vi "Control Panel No Objects.vi"(8 "error in (no error)":errorcluster) -> (0 "error out":errorcluster)   [LabVIEW 2009]
doc: "(Dynamic) A user-level application that simulates the physical front panel of the Instrument. Provide the user with buttons to manually control features of the instrument, and provide indicators of its current state."
uses:
  Global/GPIB Numbers.vi
  Microwave Amp/MicrowaveAmplifier.lvlib
panel:
  in  "Copy actual to set":bool
  in  "Populate fields with member data":bool
  in  "Read Remaining Time Delay":bool
  in  "Read Amplifier Status/Mode":bool
  in  "Standby":bool
  in  "stop":bool
  out "Mode":u16(ring) items=["SLEEP", "WARM-UP", "STANDBY", "OPERATE", "FAULT"]
  in  "Operate":bool
  in  "Read Reverse Power Out (W)":bool
  in  "Read Reverse Power Out (dBm)":bool
  in  "Read Forward Power Out (W)":bool
  in  "Read Forward Power out (dBm)":bool
  in  "Read Gain":bool
  in  "Set Gain":bool
  out "Remaining Heater Delay Time":dbl[unit]
  out "Reverse Power Out (dBm)":dbl
  out "Reverse Power Out (W)":dbl[unit]
  out "Forward Power Out (dBm)":dbl
  out "Forward Power Out (W)":dbl[unit]
  out "Gain (%)":dbl
  in  "GainSet":dbl
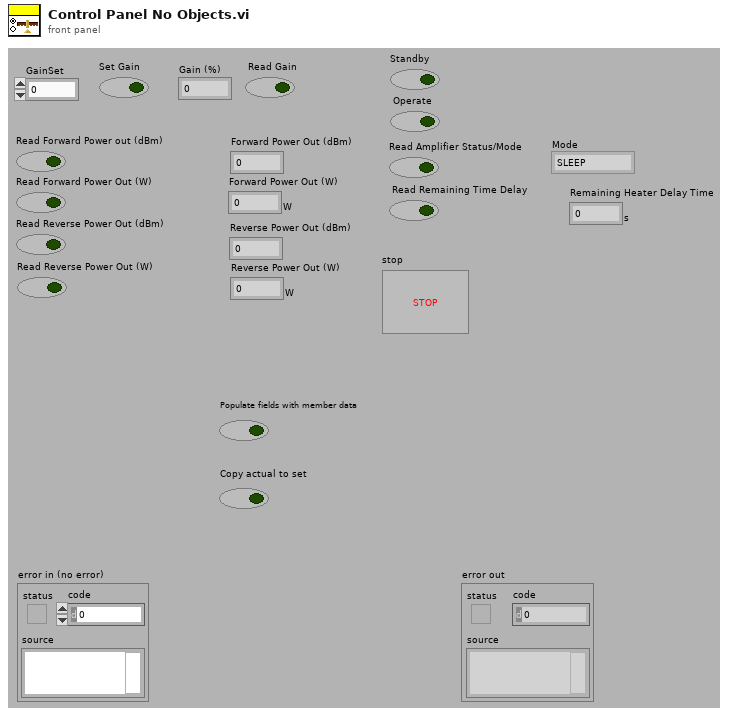
[diagram p1: front panel]
types:
  T1 = cluster{"Gain (%)":dbl, "Forward Power Out (dBm)":dbl, "Forward Power Out (W)":dbl[unit], "Reverse Power Out (dBm)":dbl, "Reverse Power Out (W)":dbl[unit], "Mode":u16, "Remaining Heater Delay Time (s)":dbl[unit]}
  T2 = typedef "GPIB Type Def.ctl" = cluster{"Name":string, "bus":dbl, "GPIB":dbl, "GPIB as string":string, "byte":i32, "VISA Resource Name":refnum<visa-resource-name>}
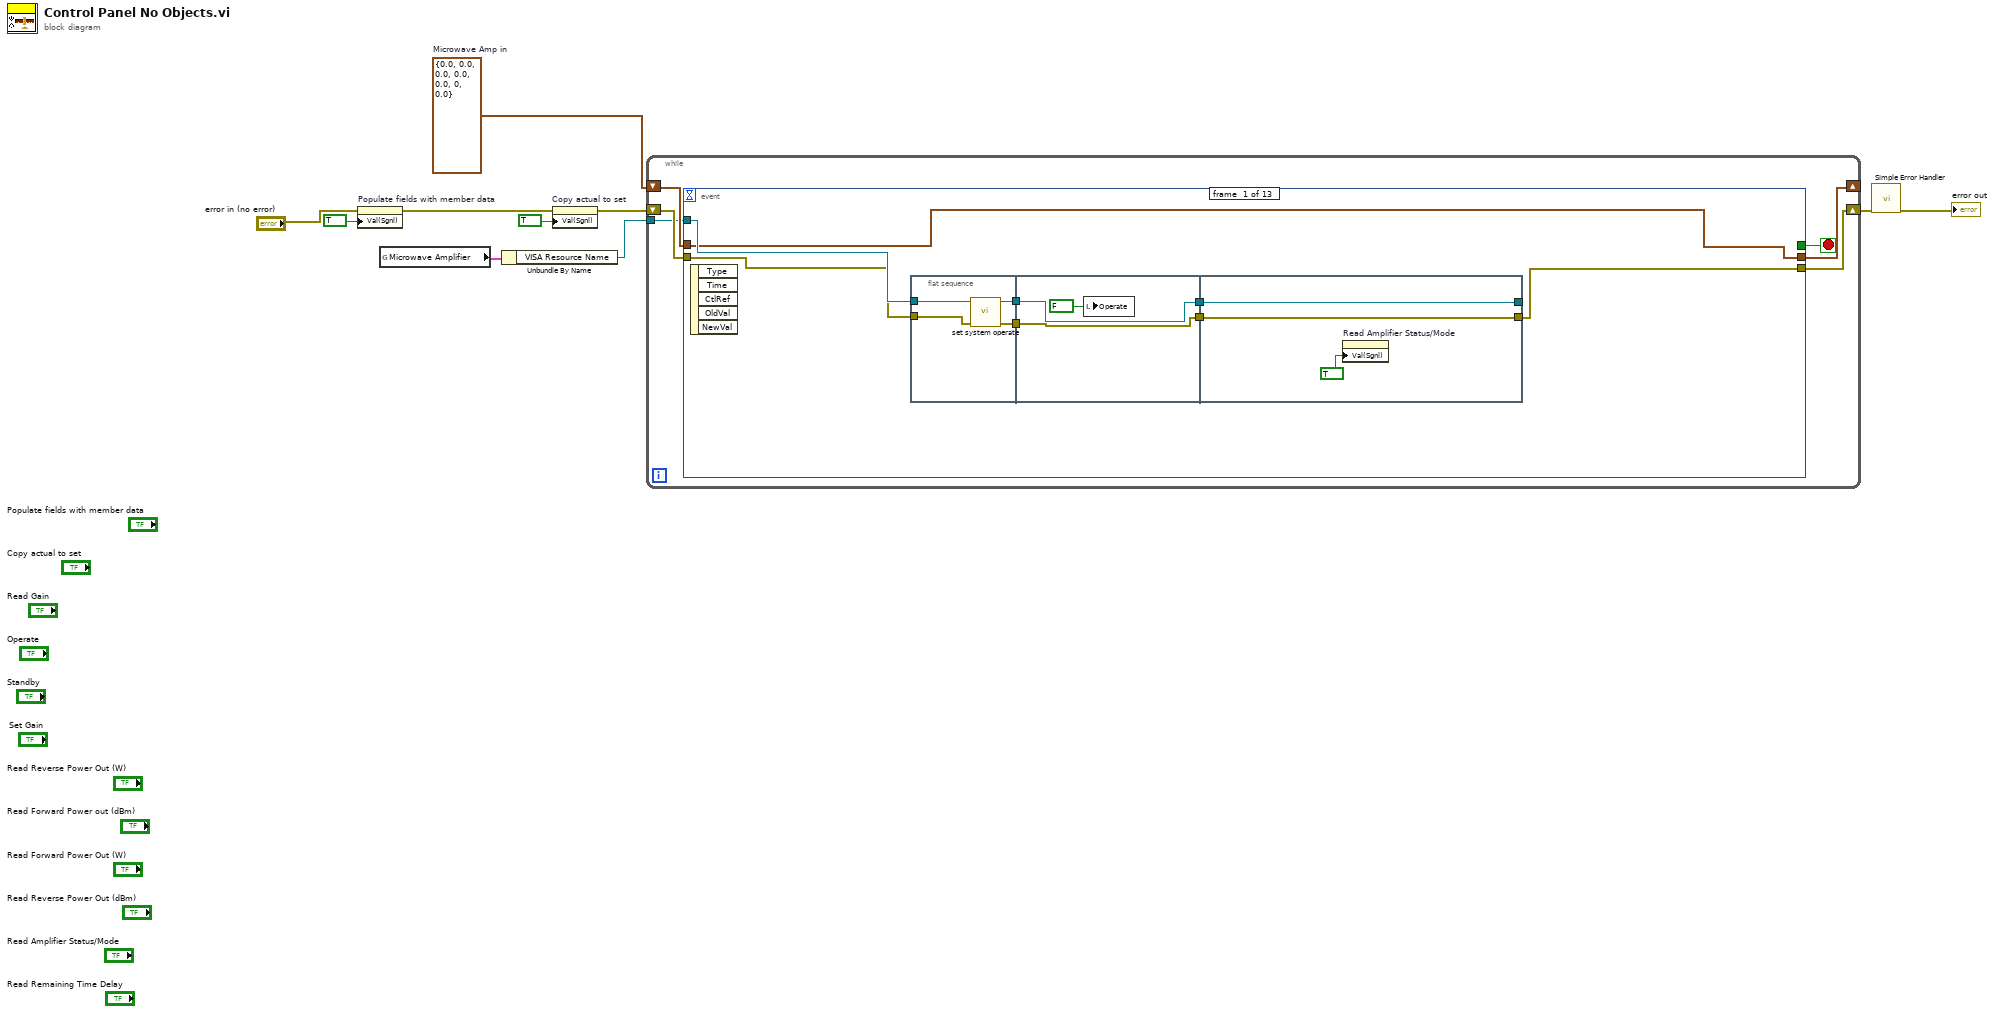
[diagram p0: block diagram]
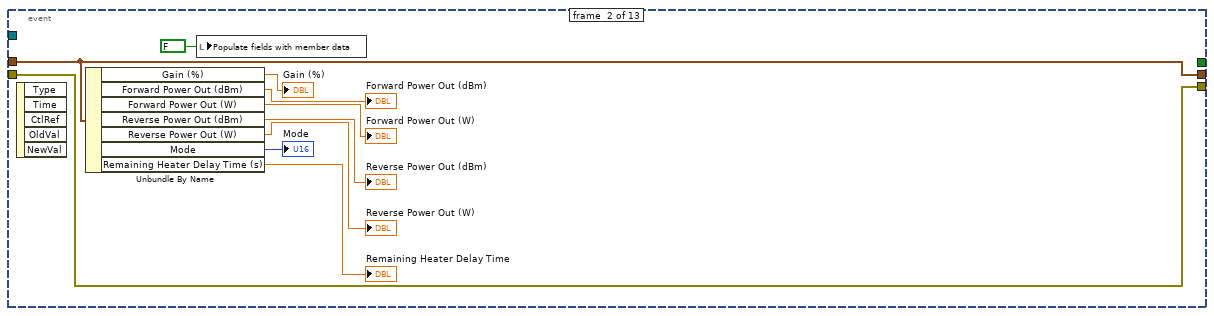
[diagram p2: hidden frame]
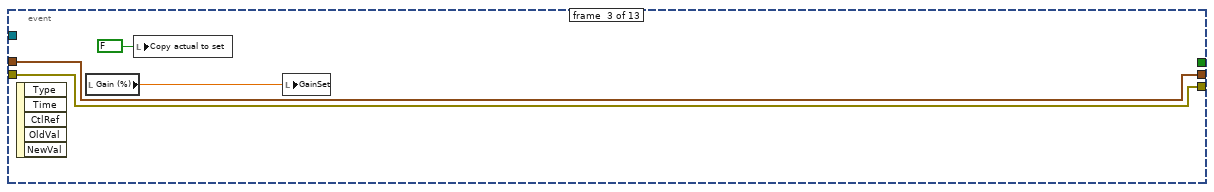
[diagram p3: hidden frame]
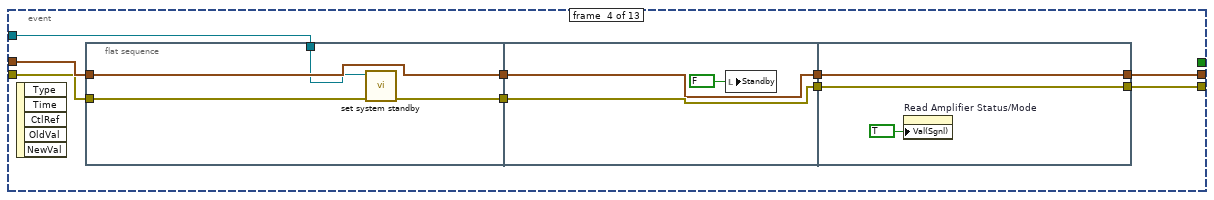
[diagram p4: hidden frame]
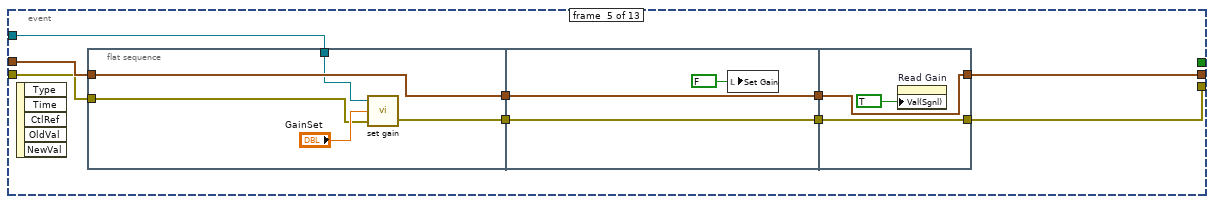
[diagram p5: hidden frame]
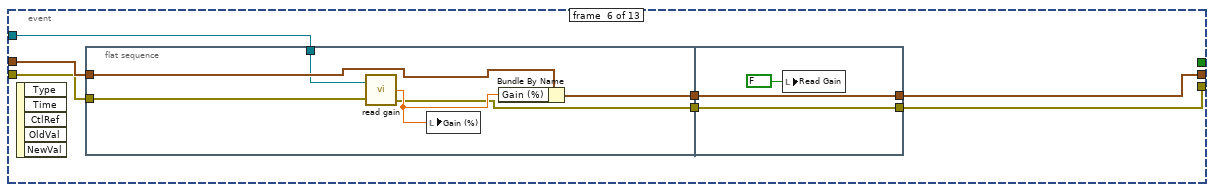
[diagram p6: hidden frame]
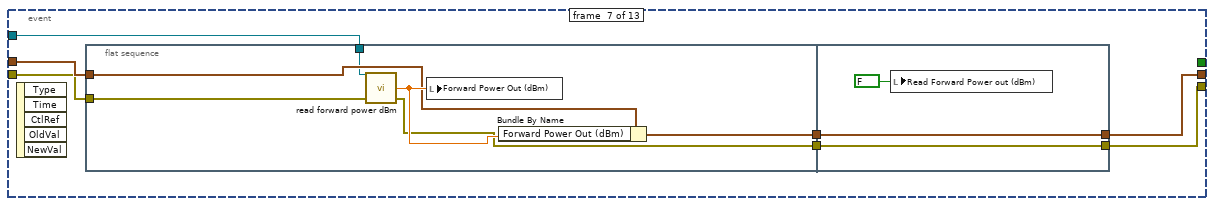
[diagram p7: hidden frame]
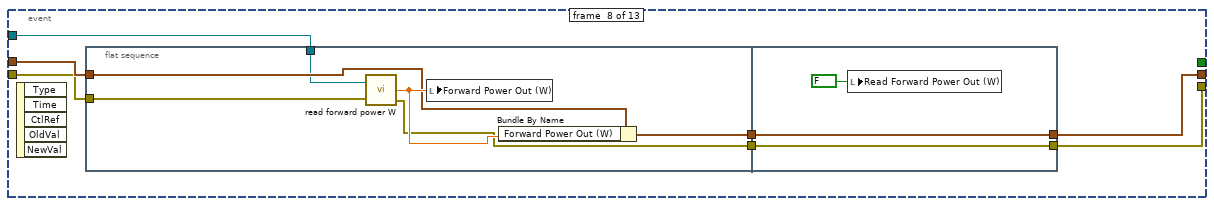
[diagram p8: hidden frame]
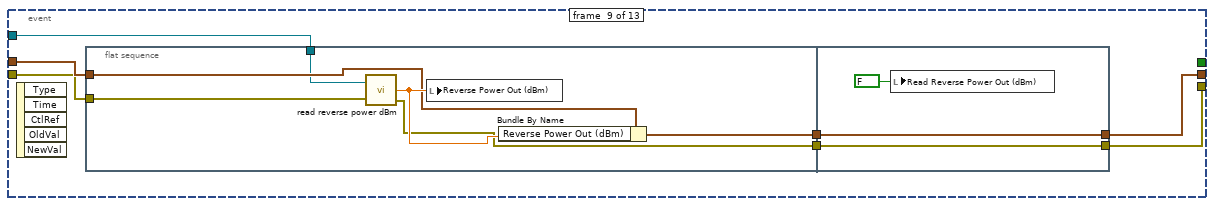
[diagram p9: hidden frame]
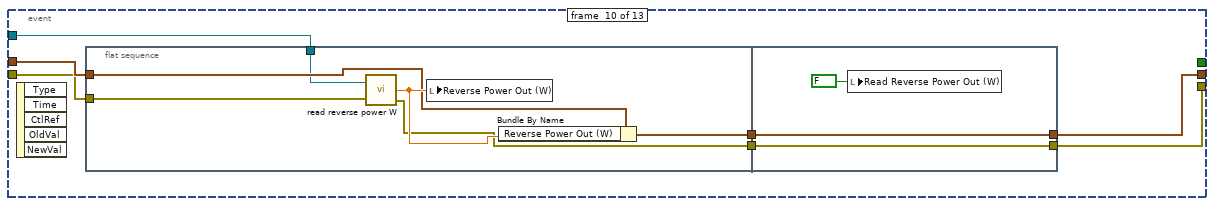
[diagram p10: hidden frame]
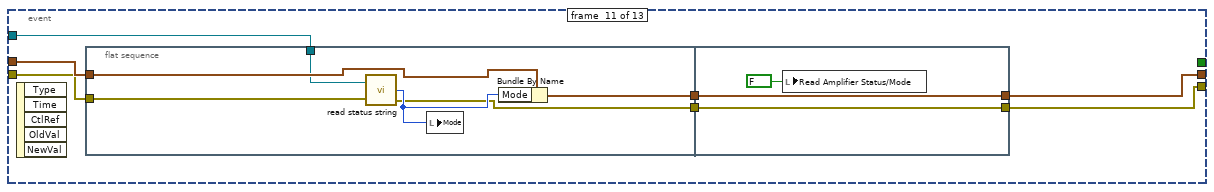
[diagram p11: hidden frame]
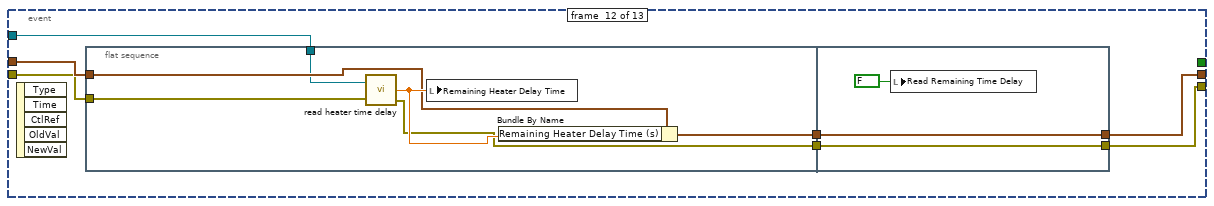
[diagram p12: hidden frame]
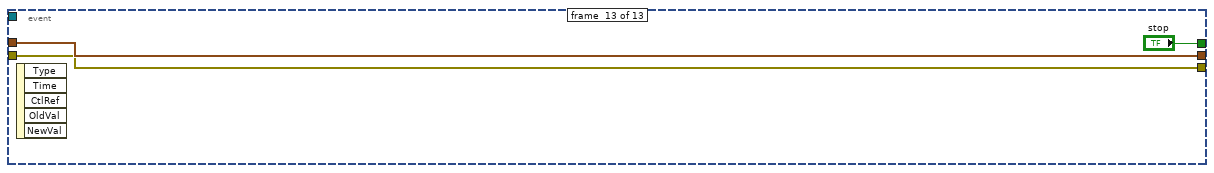
[diagram p13: hidden frame]
diagram:
  w4 = T1 {"Gain (%)"=0.0, "Forward Power Out (dBm)"=0.0, "Forward Power Out (W)"=0.0, "Reverse Power Out (dBm)"=0.0, "Reverse Power Out (W)"=0.0, "Mode"=0, "Remaining Heater Delay Time (s)"=0.0}  # Microwave Amp in
  n1 = property on="Populate fields with member data" class="Bool (strict)"(error in="error in (no error)", "Val(Sgnl)"=TRUE ("Value (Signaling)")) -> (error out=w10:errorcluster)  [unwired: 1 in, 1 out]
  n2 = global read "GPIB Numbers.vi" "Microwave Amplifier"() -> (w2:T2)
  n3 = Unbundle By Name(w2) -> ("VISA Resource Name"=w1:refnum<visa-resource-name>)
  n4 = property on="Copy actual to set" class="Bool (strict)"(error in=w10, "Val(Sgnl)"=TRUE ("Value (Signaling)")) -> (error out=w6:errorcluster)  [unwired: 1 in, 1 out]
  n5 = while {
    shift-right: [w16] -> w9
    shift-left: w6 -> [w13]
    shift-right: [w14] -> _
    shift-left: w4 -> [w12]
    tunnel: w1 -> [w11]
    stop <- w15 stop-if-true
    n6 = event shown="[12] \"stop\": Value Change" {
      selector: _ -> [_ _ _ _ _ _ _ _ _ _ _ _ _]
      dyn-events: _ -> [_ _ _ _ _ _ _ _ _ _ _ _ _]
      timeout: _ -> [_ _ _ _ _ _ _ _ _ _ _ _ _]
      tunnel: w13 -> [w19 w44 w47 w52 w73 w92 w106 w122 w138 w154 w170 w188 w200]
      tunnel: [w17 w44 w47 w56 w69 w89 w105 w121 w137 w153 w169 w185 w200] -> w16
      tunnel: [_ _ _ _ _ _ _ _ _ _ _ _ "stop"] -> w15
      tunnel: w12 -> [w18 w43 w48 w53 w74 w93 w109 w125 w141 w157 w173 w189 w201]
      tunnel: [w18 w43 w48 w54 w72 w91 w108 w124 w140 w156 w172 w187 w201] -> w14
      tunnel: w11 -> [w20 _ _ w49 w68 w88 w104 w120 w136 w152 w168 w184 _]
      event #0 {
        n7 = event-data() -> ()  [unwired: 1 in, 5 out]
        n8 = flat-sequence {
          tunnel: [w28] -> w24
          tunnel: [w27] -> w23
          tunnel: w19 -> [w26]
          tunnel: w20 -> [w25]
          tunnel: w24 -> [w30]
          tunnel: w23 -> [w29]
          tunnel: [w30] -> w22
          tunnel: [w29] -> w21
          tunnel: [w33] -> w17
          tunnel: [w34] -> _
          tunnel: w22 -> [w34]
          tunnel: w21 -> [w33]
          frame #0 {
            n9 = call "set system operate.vi"("error in (no error)"=w26, "VISA resource name"=w25) -> ("error out"=w27:errorcluster, "VISA resource name out"=w28:refnum<visa-resource-name>)  [unwired: 8 in]
          }
          frame #1 {
            n10 = local write "Operate"(FALSE ("Operate")) -> ()
          }
          frame #2 {
            n11 = property on="Read Amplifier Status/Mode" class="Bool (strict)"("Val(Sgnl)"=TRUE ("Value (Signaling)")) -> ()  [unwired: 2 in, 2 out]
          }
        }
      }
      event #1 {
        n12 = event-data() -> ()  [unwired: 1 in, 5 out]
        n13 = Unbundle By Name(w43) -> ("Gain (%)"=→"Gain (%)":dbl, "Forward Power Out (dBm)"=→"Forward Power Out (dBm)":dbl, "Forward Power Out (W)"=→"Forward Power Out (W)":dbl[unit], "Reverse Power Out (dBm)"=→"Reverse Power Out (dBm)":dbl, "Reverse Power Out (W)"=→"Reverse Power Out (W)":dbl[unit], "Mode"=→"Mode":u16, "Remaining Heater Delay Time (s)"=→"Remaining Heater Delay Time":dbl[unit])
        n14 = local write "Populate fields with member data"(FALSE ("Populate fields with member data")) -> ()
      }
      event #2 {
        n15 = event-data() -> ()  [unwired: 1 in, 5 out]
        n16 = local read "Gain (%)"() -> (w45:dbl)
        n17 = local write "Copy actual to set"(FALSE ("Copy actual to set")) -> ()
        n18 = local write "GainSet"(w45) -> ()
      }
      event #3 {
        n19 = event-data() -> ()  [unwired: 1 in, 5 out]
        n20 = flat-sequence {
          tunnel: [w61] -> w57
          tunnel: [w60] -> w55
          tunnel: w53 -> [w60]
          tunnel: w52 -> [w59]
          tunnel: w49 -> [w58]
          tunnel: w57 -> [w63]
          tunnel: w55 -> [w62]
          tunnel: [w63] -> w51
          tunnel: [w62] -> w50
          tunnel: [w66] -> w54
          tunnel: [w67] -> w56
          tunnel: w51 -> [w67]
          tunnel: w50 -> [w66]
          frame #0 {
            n21 = call "set system standby.vi"("error in (no error)"=w59, "VISA resource name"=w58) -> ("error out"=w61:errorcluster)  [unwired: 8 in, 1 out]
          }
          frame #1 {
            n22 = local write "Standby"(FALSE ("Operate")) -> ()
          }
          frame #2 {
            n23 = property on="Read Amplifier Status/Mode" class="Bool (strict)"("Val(Sgnl)"=TRUE ("Value (Signaling)")) -> ()  [unwired: 2 in, 2 out]
          }
        }
      }
      event #4 {
        n24 = event-data() -> ()  [unwired: 1 in, 5 out]
        n25 = flat-sequence {
          tunnel: [w80] -> w76
          tunnel: w74 -> [w79]
          tunnel: w73 -> [w78]
          tunnel: [w79] -> w70
          tunnel: w68 -> [w77]
          tunnel: w76 -> [w83]
          tunnel: [w83] -> w75
          tunnel: [w82] -> w71
          tunnel: w70 -> [w82]
          tunnel: [w87] -> w69
          tunnel: w75 -> [w87]
          tunnel: [w85] -> w72
          tunnel: w71 -> [w85]
          frame #0 {
            n26 = call "set gain.vi"("error in (no error)"=w78, "Gain"="GainSet", "VISA resource name"=w77) -> ("error out"=w80:errorcluster)  [unwired: 1 out]
          }
          frame #1 {
            n27 = local write "Set Gain"(FALSE ("Set Gain")) -> ()
          }
          frame #2 {
            n28 = property on="Read Gain" class="Bool (strict)"("Val(Sgnl)"=TRUE ("Value (Signaling)")) -> ()  [unwired: 2 in, 2 out]
          }
        }
      }
      event #5 {
        n29 = event-data() -> ()  [unwired: 1 in, 5 out]
        n30 = flat-sequence {
          tunnel: [w98] -> w94
          tunnel: w93 -> [w96]
          tunnel: w92 -> [w97]
          tunnel: [w99] -> w90
          tunnel: w88 -> [w95]
          tunnel: [w102] -> w89
          tunnel: w94 -> [w102]
          tunnel: [w101] -> w91
          tunnel: w90 -> [w101]
          frame #0 {
            n31 = call "read gain.vi"("VISA resource name"=w95, "error in (no error)"=w97) -> ("Gain (%)"=w100:dbl, "error out"=w98:errorcluster)  [unwired: 1 out]
            n32 = local write "Gain (%)"(w100) -> ()
            n33 = Bundle By Name(cluster=w96, "Gain (%)"=w100) -> (w99:T1)
          }
          frame #1 {
            n34 = local write "Read Gain"(FALSE ("Read Gain")) -> ()
          }
        }
      }
      event #6 {
        n35 = event-data() -> ()  [unwired: 1 in, 5 out]
        n36 = flat-sequence {
          tunnel: [w112] -> w110
          tunnel: w109 -> [w113]
          tunnel: [w115] -> w107
          tunnel: w106 -> [w114]
          tunnel: w104 -> [w111]
          tunnel: [w119] -> w105
          tunnel: w110 -> [w119]
          tunnel: [w117] -> w108
          tunnel: w107 -> [w117]
          frame #0 {
            n37 = call "read forward power dBm.vi"("error in (no error)"=w114, "VISA resource name"=w111) -> ("error out"=w112:errorcluster, "forward power (dBm)"=w116:dbl)  [unwired: 1 in, 1 out]
            n38 = local write "Forward Power Out (dBm)"(w116) -> ()
            n39 = Bundle By Name(cluster=w113, "Forward Power Out (dBm)"=w116) -> (w115:T1)
          }
          frame #1 {
            n40 = local write "Read Forward Power out (dBm)"(FALSE ("Read Forward Power out (dBm)")) -> ()
          }
        }
      }
      event #7 {
        n41 = event-data() -> ()  [unwired: 1 in, 5 out]
        n42 = flat-sequence {
          tunnel: [w130] -> w126
          tunnel: w125 -> [w128]
          tunnel: [w131] -> w123
          tunnel: w122 -> [w129]
          tunnel: w120 -> [w127]
          tunnel: [w135] -> w121
          tunnel: w126 -> [w135]
          tunnel: [w133] -> w124
          tunnel: w123 -> [w133]
          frame #0 {
            n43 = call "read forward power W.vi"("VISA resource name"=w127, "error in (no error)"=w129) -> ("foward power (W)"=w132:dbl[unit], "error out"=w130:errorcluster)  [unwired: 1 out]
            n44 = local write "Forward Power Out (W)"(w132) -> ()
            n45 = Bundle By Name(cluster=w128, "Forward Power Out (W)"=w132) -> (w131:T1)
          }
          frame #1 {
            n46 = local write "Read Forward Power Out (W)"(FALSE ("Read Forward Power Out (W)")) -> ()
          }
        }
      }
      event #8 {
        n47 = event-data() -> ()  [unwired: 1 in, 5 out]
        n48 = flat-sequence {
          tunnel: [w146] -> w142
          tunnel: w141 -> [w144]
          tunnel: [w147] -> w139
          tunnel: w138 -> [w145]
          tunnel: w136 -> [w143]
          tunnel: [w150] -> w137
          tunnel: w142 -> [w150]
          tunnel: [w149] -> w140
          tunnel: w139 -> [w149]
          frame #0 {
            n49 = call "read reverse power dBm.vi"("VISA resource name"=w143, "error in (no error)"=w145) -> ("reverse power (dBm)"=w148:dbl, "error out"=w146:errorcluster)  [unwired: 1 out]
            n50 = local write "Reverse Power Out (dBm)"(w148) -> ()
            n51 = Bundle By Name(cluster=w144, "Reverse Power Out (dBm)"=w148) -> (w147:T1)
          }
          frame #1 {
            n52 = local write "Read Reverse Power Out (dBm)"(FALSE ("Read Reverse Power Out (dBm)")) -> ()
          }
        }
      }
      event #9 {
        n53 = event-data() -> ()  [unwired: 1 in, 5 out]
        n54 = flat-sequence {
          tunnel: [w161] -> w158
          tunnel: w157 -> [w160]
          tunnel: [w164] -> w155
          tunnel: w154 -> [w162]
          tunnel: w152 -> [w159]
          tunnel: [w166] -> w153
          tunnel: w158 -> [w166]
          tunnel: [w165] -> w156
          tunnel: w155 -> [w165]
          frame #0 {
            n55 = call "read reverse power W.vi"("VISA resource name"=w159, "error in (no error)"=w162) -> ("Reverse Power (W)"=w163:dbl[unit], "error out"=w161:errorcluster)  [unwired: 1 out]
            n56 = local write "Reverse Power Out (W)"(w163) -> ()
            n57 = Bundle By Name(cluster=w160, "Reverse Power Out (W)"=w163) -> (w164:T1)
          }
          frame #1 {
            n58 = local write "Read Reverse Power Out (W)"(FALSE ("Read Reverse Power Out (W)")) -> ()
          }
        }
      }
      event #10 {
        n59 = event-data() -> ()  [unwired: 1 in, 5 out]
        n60 = flat-sequence {
          tunnel: [w177] -> w174
          tunnel: w173 -> [w176]
          tunnel: [w180] -> w171
          tunnel: w170 -> [w178]
          tunnel: w168 -> [w175]
          tunnel: [w183] -> w169
          tunnel: w174 -> [w183]
          tunnel: [w181] -> w172
          tunnel: w171 -> [w181]
          frame #0 {
            n61 = call "read status string.vi"("VISA resource name"=w175, "error in (no error)"=w178) -> ("Mode"=w179:u16, "error out"=w177:errorcluster)  [unwired: 1 out]
            n62 = local write "Mode"(w179) -> ()
            n63 = Bundle By Name(cluster=w176, "Mode"=w179) -> (w180:T1)
          }
          frame #1 {
            n64 = local write "Read Amplifier Status/Mode"(FALSE ("Read Amplifier Status")) -> ()
          }
        }
      }
      event #11 {
        n65 = event-data() -> ()  [unwired: 1 in, 5 out]
        n66 = flat-sequence {
          tunnel: [w194] -> w190
          tunnel: w189 -> [w193]
          tunnel: w188 -> [w192]
          tunnel: [w195] -> w186
          tunnel: w184 -> [w191]
          tunnel: [w199] -> w185
          tunnel: w190 -> [w199]
          tunnel: [w197] -> w187
          tunnel: w186 -> [w197]
          frame #0 {
            n67 = call "read heater time delay.vi"("VISA resource name"=w191, "error in (no error)"=w192) -> ("Heater delay time (s)"=w196:dbl[unit], "error out"=w194:errorcluster)  [unwired: 1 out]
            n68 = local write "Remaining Heater Delay Time"(w196) -> ()
            n69 = Bundle By Name(cluster=w193, "Remaining Heater Delay Time (s)"=w196) -> (w195:T1)
          }
          frame #1 {
            n70 = local write "Read Remaining Time Delay"(FALSE ("Read Remaining Time Delay")) -> ()
          }
        }
      }
      event #12 {
        n71 = event-data() -> ()  [unwired: 1 in, 5 out]
      }
    }
  }
  n72 = call <vilib>:"Simple Error Handler.vi"("error in (no error)"=w9) -> ("error out"=→"error out":errorcluster)  [unwired: 1 in, 7 out]
